vi "Untitled 4 (SubVI).vi"(0 "x 19":dbl, 1 "x 18":dbl, 2 "x 17":dbl, 3 "x 16":dbl, 4 "x 15":dbl, 6 "x 20":dbl, 7 "x 14":dbl, 8 "x 4":dbl, 9 "x 13":dbl) -> (10 "x 3":dbl, 11 "x 12":dbl, 12 "x 5":dbl, 13 "x 11":dbl, 14 "x 6":dbl, 15 "x 7":dbl, 16 "x 8":dbl, 17 "x 9":dbl, 18 "x 10":dbl)   [LabVIEW 2013]
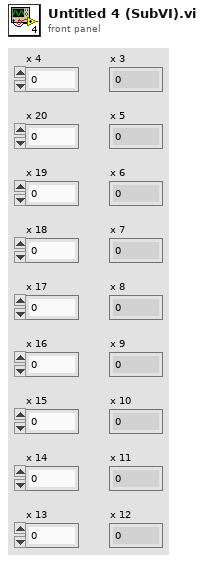
[diagram p1: front panel]
types:
  T1 = cluster{"x 20":dbl, "x 19":dbl, "x 18":dbl, "x 17":dbl, "x 16":dbl, "x 15":dbl, "x 14":dbl, "x 13":dbl}
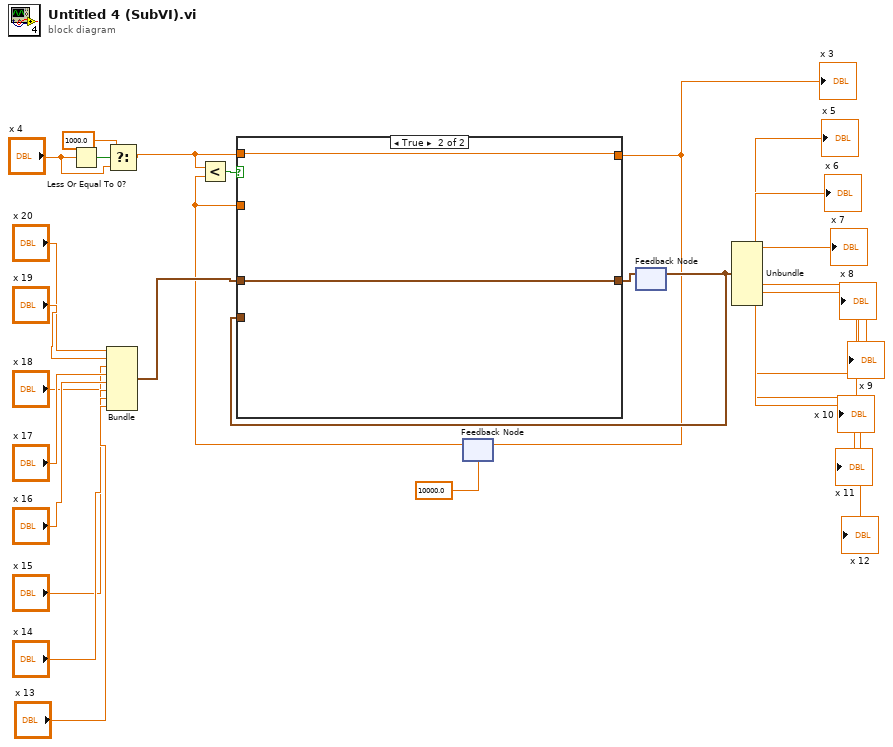
[diagram p0: block diagram]
diagram:
  n1 = Less Or Equal To 0?(x="x 4") -> (x <= 0?=w5:bool)
  n2 = Bundle("x 20"="x 20", "x 19"="x 19", "x 18"="x 18", "x 17"="x 17", "x 16"="x 16", "x 15"="x 15", "x 14"="x 14", "x 13"="x 13") -> (w17:T1)  [unwired: 1 in]
  n3 = Select(t=1000.0, s=w5, f="x 4") -> (s? t:f=w2:dbl)
  n4 = feedback #1(10000.0 ("x")) -> (w8:dbl)
  n5 = Less?(x=w2, y=w8) -> (x < y?=w6:bool)
  n6 = feedback #2() -> (w19:T1)  [unwired: 1 in]
  n7 = case shown="True" w6 {
    tunnel: w2 -> [_ w31]
    tunnel: [w29 w31] -> w7
    tunnel: w8 -> [w29 _]
    tunnel: w17 -> [_ w30]
    tunnel: [w28 w30] -> w18
    tunnel: w19 -> [w28 _]
    frame False {
    }
    frame True {
    }
  }
  "x 3" <- w7
  n8 = feedback-in #1(w7) -> ()
  n9 = feedback-in #2(w18) -> ()
  n10 = Unbundle(w19) -> ("x 20"=→"x 5":dbl, "x 19"=→"x 6":dbl, "x 18"=→"x 7":dbl, "x 17"=→"x 8":dbl, "x 16"=→"x 9":dbl, "x 15"=→"x 10":dbl, "x 14"=→"x 11":dbl, "x 13"=→"x 12":dbl)
